vi "TagbusToCluster.vi"(8 "error in":errorcluster, 9 "index cluster":T1, 11 "tag bus in":T3) -> (0 "error out":errorcluster, 2 "cluster":T2, 3 "tag bus out":T3)   [LabVIEW 2013]
uses:
  <vilib>/NI/Tag Bus/table/data table.ctl
  Controls/SampleControl.ctl
  Controls/IndexCluster.ctl
  <vilib>/NI/Tag Bus/table/data polymorphs/read one/read Array of Double.vi
  <vilib>/NI/Tag Bus/table/data polymorphs/read one/read Boolean.vi
  <vilib>/NI/Tag Bus/table/data polymorphs/read one/read Double.vi
  <vilib>/NI/Tag Bus/table/data polymorphs/read one/read String.vi
  <vilib>/NI/Tag Bus/table/data table.lvlib
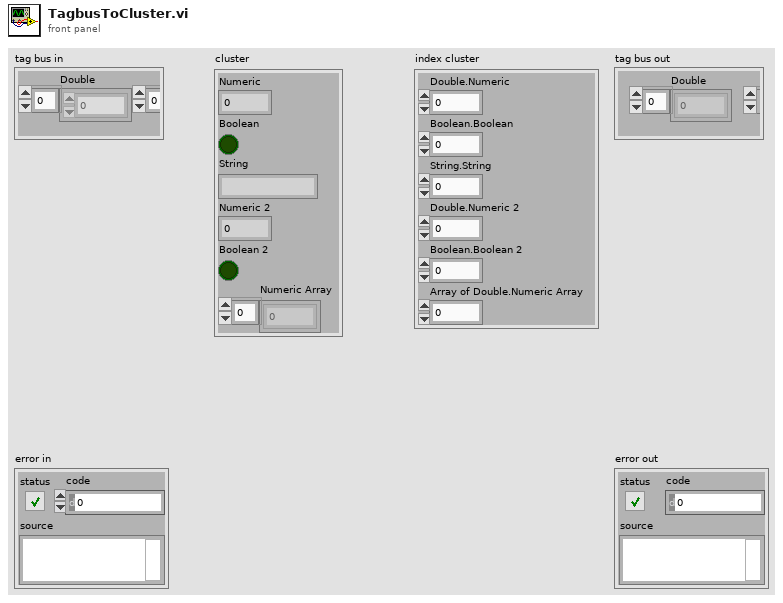
[diagram p1: front panel]
types:
  T1 = typedef "IndexCluster.ctl" = cluster{"Double.Numeric":i32, "Boolean.Boolean":i32, "String.String":i32, "Double.Numeric 2":i32, "Boolean.Boolean 2":i32, "Array of Double.Numeric Array":i32}
  T2 = typedef "SampleControl.ctl" = cluster{"Numeric":dbl, "Boolean":bool, "String":string, "Numeric 2":dbl, "Boolean 2":bool, "Numeric Array":dbl[]}
  T3 = typedef "tag bus.lvlib/data table.lvlib/data table.ctl" = cluster{"Double":dbl[], "Single":sgl[], "I64":i64[], "I32":i32[], "I16":i16[], "I8":i8[], "U64":u64[], "U32":u32[], "U16":u16[], "U8":u8[], "Boolean":bool[], "String":string[], "Array of Double":cluster{"DBL Array":dbl[]}[], "Array of Single":cluster{"SGL Array":sgl[]}[], "Array of I64":cluster{"I64 Array":i64[]}[], "Array of I32":cluster{"I32 Array":i32[]}[], "Array of I16":cluster{"I16 Array":i16[]}[], "Array of I8":cluster{"I8 Array":i8[]}[], "Array of U64":cluster{"U64 Array":u64[]}[], "Array of U32":cluster{"U32 Array":u32[]}[], "Array of U16":cluster{"U16 Array":u16[]}[], "Array of U8":cluster{"U8 Array":u8[]}[], "Array of Boolean":cluster{"Boolean Array":bool[]}[], "Array of String":cluster{"String Array":string[]}[]}
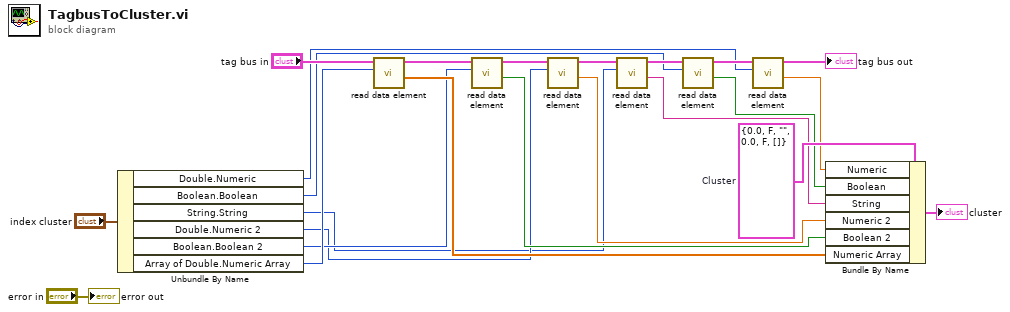
[diagram p0: block diagram]
diagram:
  w22 = T2 {"Numeric"=0.0, "Boolean"=FALSE, "String"="", "Numeric 2"=0.0, "Boolean 2"=FALSE, "Numeric Array"=[]}  # Cluster
  n1 = Unbundle By Name("index cluster") -> ("Double.Numeric"=w3:i32, "Boolean.Boolean"=w6:i32, "String.String"=w9:i32, "Double.Numeric 2"=w12:i32, "Boolean.Boolean 2"=w15:i32, "Array of Double.Numeric Array"=w18:i32)
  n2 = call-poly <vilib>:"read data element.vi"("index"=w18, "data table in"="tag bus in") -> ("value"=w19:dbl[], "data table out"=w17:T3)  [unwired: 8 in]
  n3 = call-poly <vilib>:"read data element.vi"("index"=w15, "data table in"=w17) -> ("value"=w16:bool, "data table out"=w14:T3)  [unwired: 8 in]
  n4 = call-poly <vilib>:"read data element.vi"("index"=w12, "data table in"=w14) -> ("value"=w13:dbl, "data table out"=w11:T3)  [unwired: 8 in]
  n5 = call-poly <vilib>:"read data element.vi"("index"=w9, "data table in"=w11) -> ("value"=w10:string, "data table out"=w8:T3)  [unwired: 8 in]
  n6 = call-poly <vilib>:"read data element.vi"("index"=w6, "data table in"=w8) -> ("value"=w7:bool, "data table out"=w5:T3)  [unwired: 8 in]
  n7 = call-poly <vilib>:"read data element.vi"("index"=w3, "data table in"=w5) -> ("value"=w4:dbl, "data table out"=→"tag bus out":T3)  [unwired: 8 in]
  n8 = Bundle By Name(cluster=w22, "Numeric"=w4, "Boolean"=w7, "String"=w10, "Numeric 2"=w13, "Boolean 2"=w16, "Numeric Array"=w19) -> (→"cluster":T2)
  "error out" <- "error in"
